vi "TB-Post Slack Messages.vi"(0 "Slack":T1, 7 "Message":string, 9 "error notification (F)":bool, 11 "error in (no error)":errorcluster) -> (15 "error out":errorcluster)   [LabVIEW 2020]
uses:
  Typedefs/TB-Slack State.ctl
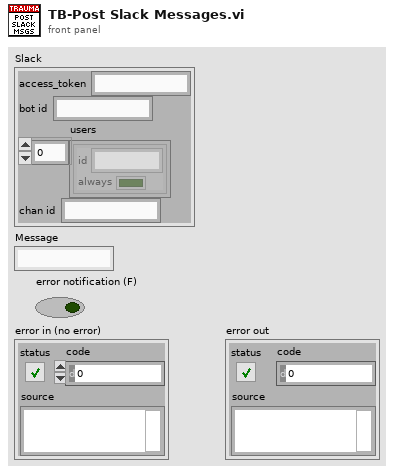
[diagram p1: front panel]
types:
  T1 = typedef "TB-Slack State.ctl" = cluster{"access_token":string, "bot id":string, "users":cluster{"id":string, "always":bool}[], "chan id":string}
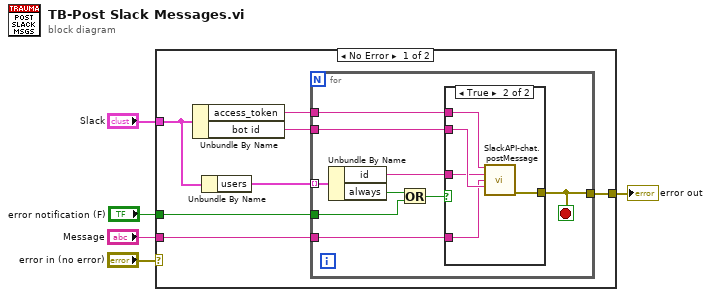
[diagram p0: block diagram]
diagram:
  n1 = case shown="No Error" "error in (no error)" {
    selector: "error in (no error)" -> [_ w27]
    tunnel: [w12 w27] -> w2
    tunnel: "Slack" -> [w8 _]
    tunnel: "Message" -> [w9 _]
    tunnel: "error notification (F)" -> [w6 _]
    frame No Error {
      n2 = Unbundle By Name(w8) -> ("access_token"=w11:string, "bot id"=w10:string)
      n3 = Unbundle By Name(w8) -> ("users"=w7:cluster{"id":string, "always":bool}[])
      n4 = for {
        tunnel: w11 -> [w21]
        tunnel: [w19] -> w12
        tunnel: w10 -> [w20]
        tunnel: w7 -> [w17] mode=indexing
        tunnel: w9 -> [w18]
        tunnel: w6 -> [w13]
        stop <- w19 stop-if-true
        n5 = Unbundle By Name(w17) -> ("id"=w16:string, "always"=w14:bool)
        n6 = Or(x=w14, y=w13) -> (x .or. y?=w15:bool)
        n7 = case shown="True" w15 {
          tunnel: w21 -> [_ w26]
          tunnel: w20 -> [_ w25]
          tunnel: [_ w24] -> w19
          tunnel: w18 -> [_ w23]
          tunnel: w16 -> [_ w22]
          frame False {
          }
          frame True {
            n8 = call "SlackAPI-chat.postMessage.vi"("access_token"=w26, "user ID"=w22, "message"=w23, "username"=w25) -> ("error out"=w24:errorcluster)  [unwired: 11 in]
          }
        }
      }
    }
    frame Error {
    }
  }
  "error out" <- w2
